vi "TP 3.3.vi"() -> ()   [LabVIEW 2013]
uses:
  <vilib>/sound2/lvsound2.llb/Sound Input Read (DBL).vi
panel:
  in  "Cluster":T1={"Sample rate"=54100.0, "N channels"=1.0, " bits per sample"=16.0}
  out "Waveform Graph":dbl[](graph)
  in  "Buffer de lectura":dbl=11025.0
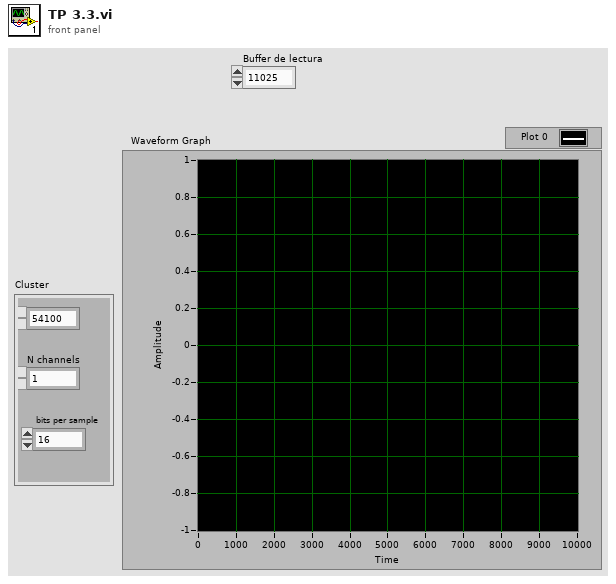
[diagram p1: front panel]
types:
  T1 = cluster{"Sample rate":dbl, "N channels":dbl, " bits per sample":dbl}
  T2 = typedef "Sound Input Task ID.ctl" = u32
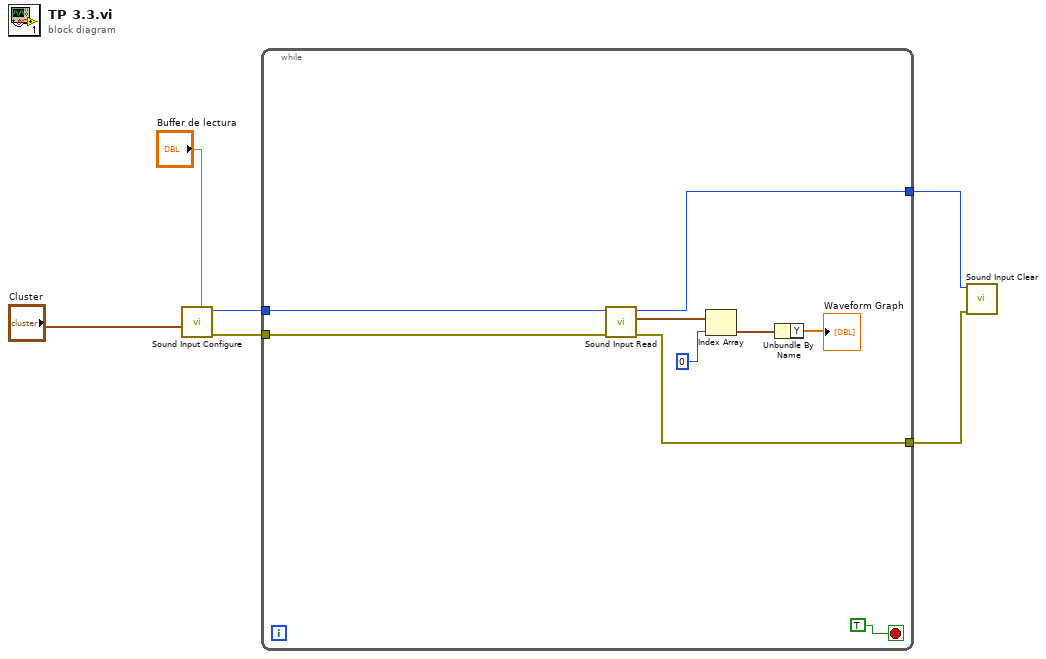
[diagram p0: block diagram]
diagram:
  n1 = call <vilib>:"Sound Input Configure.vi"("number of samples/ch"="Buffer de lectura", "sound format"="Cluster") -> ("error out"=w4:errorcluster, "task ID"=w5:T2)  [unwired: 8 in]
  n2 = while {
    tunnel: w5 -> [w11]
    tunnel: w4 -> [w10]
    tunnel: [w9] -> w2
    tunnel: [w8] -> w1
    stop <- TRUE stop-if-true
    n3 = call-poly <vilib>:"Sound Input Read.vi"("error in (no error)"=w10, "task ID"=w11) -> ("error out"=w8:errorcluster, "data"=w15:waveform(dbl)[], "task ID out"=w9:T2)  [unwired: 7 in]
    n4 = Index Array(array=w15, index=0) -> (element=w13:waveform(dbl))
    n5 = Unbundle By Name(w13) -> ("Y"=→"Waveform Graph":dbl[])
  }
  n6 = call <vilib>:"Sound Input Clear.vi"("error in (no error)"=w1, "task ID"=w2) -> ()  [unwired: 9 in, 1 out]
